vi "CalculateFloatA.vi"(9 "sinHalfTheta":dbl, 10 "HalfTheta":dbl, 11 "t":dbl) -> (3 "FloatRatioA":dbl)   [LabVIEW 2016]
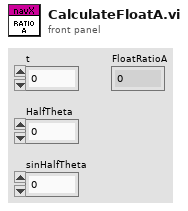
[diagram p1: front panel]
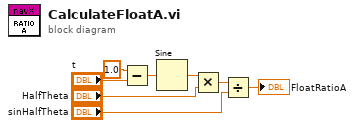
[diagram p0: block diagram]
diagram:
  n1 = Subtract(x=1.0, y="t") -> (x-y=w2:dbl)
  n2 = Sine(x=w2) -> (sin(x)=w4:dbl)
  n3 = Multiply(x=w4, y="HalfTheta") -> (x*y=w6:dbl)
  n4 = Divide(x=w6, y="sinHalfTheta") -> (x/y=→"FloatRatioA":dbl)
